vi "Get global var file or mem.vi"(8 "error in (no error)":errorcluster, 9 "Config file path name":string="use default", 10 "Key Name":string="test_pc_name", 11 "Section Name":string="general") -> (0 "error out":errorcluster, 1 "Yes?":bool, 2 "KeyFound?":bool, 3 "Key data from file":string)   [LabVIEW 2013]
doc: "Gets key data from global.ini file in exe directory"
uses:
  <vilib>/Utility/error.llb/whitespace.ctl
  Test Globals/Global 1.vi
panel:
  out "Boolean":bool
  out "Using memory?":bool
  out "Info block":string
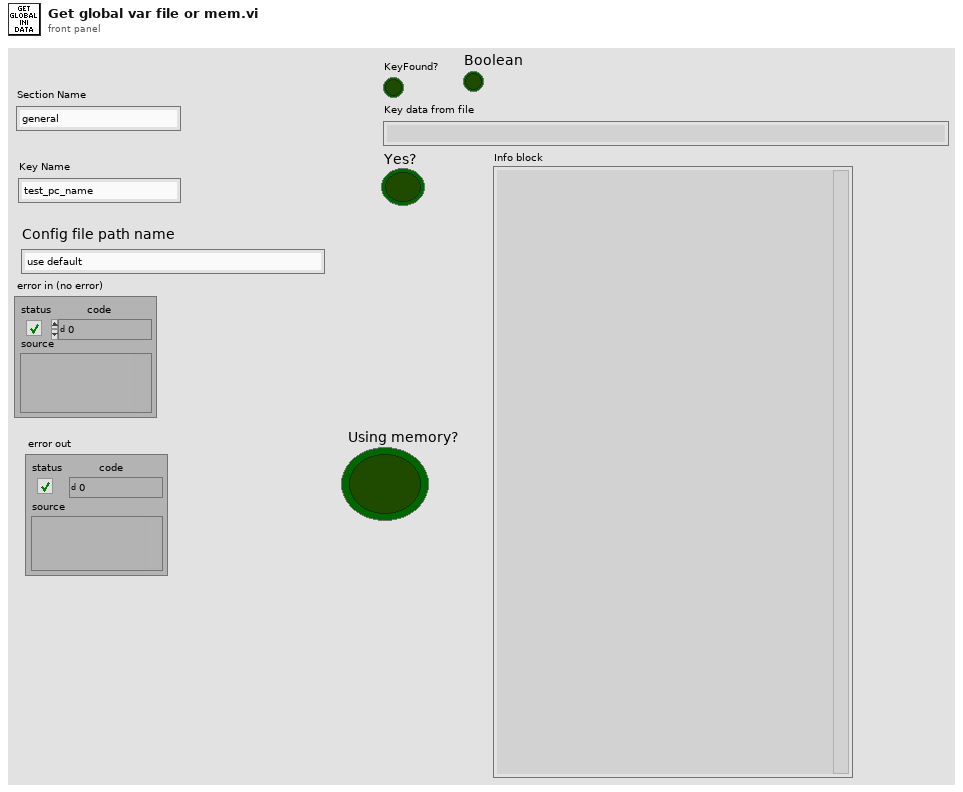
[diagram p1: front panel]
types:
  T1 = cluster{"Test folder":string, "Top level":string, "Main":string, "Test report":string, "Work order qty":string, "Work order meid":string, "Work order imei":string, "Master meid imei list":string, "Master test data":string, "ZPL label info":string, "Pictures":string, "Setup info":string, "Work order":string, "Tests folder":string, "Tests steps folder":string, "Config folder":string, "Verizon Upload file":string, "Job data file":string, "Station globals":string, "Post test info":string}
  T2 = typedef "whitespace.ctl" = u16
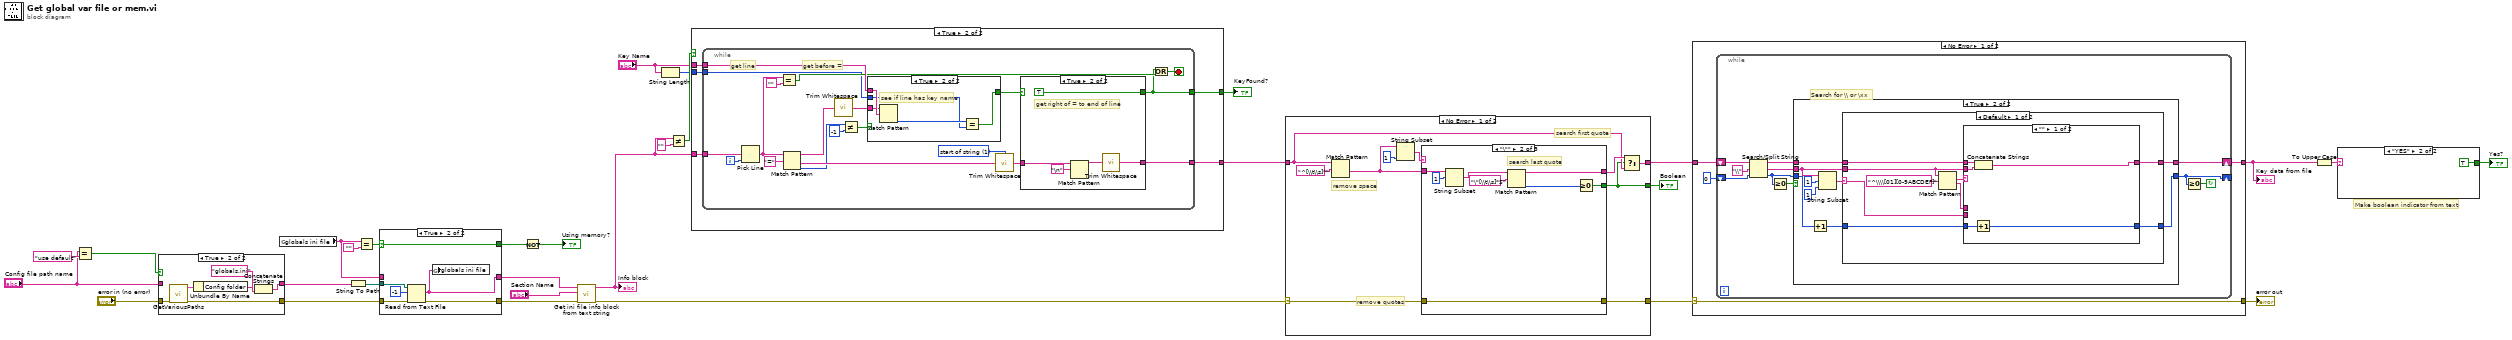
[diagram p0: block diagram]
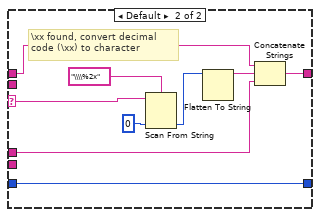
[diagram p4: hidden frame]
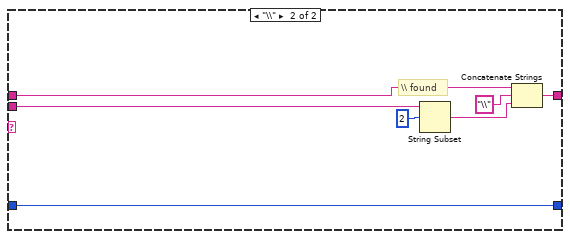
[diagram p5: hidden frame]
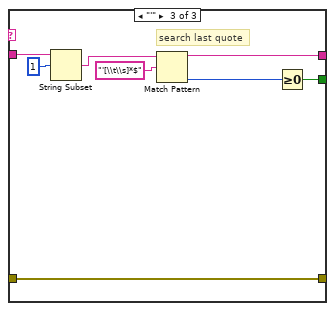
[diagram p8: hidden frame]
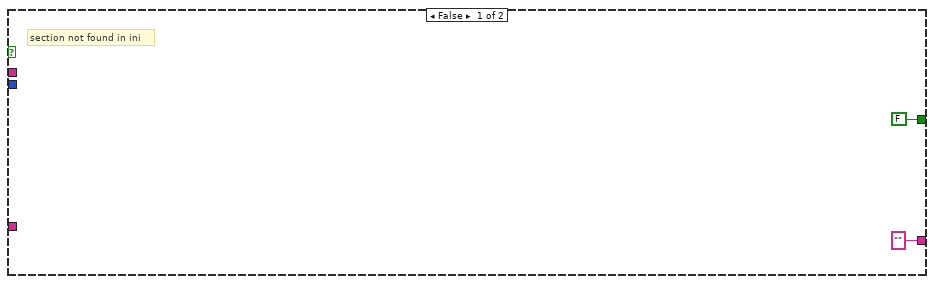
[diagram p10: hidden frame]
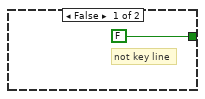
[diagram p11: hidden frame]
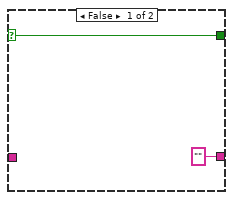
[diagram p12: hidden frame]
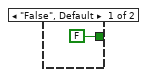
[diagram p14: hidden frame]
diagram:
  # "Make boolean indicator from text"
  n1 = Equal?(x="Config file path name", y="use default") -> (x = y?=w2:bool)
  n2 = case shown="True" w2 {
    tunnel: "error in (no error)" -> [w31 w35]
    tunnel: [w32 w34] -> w29
    tunnel: [w31 w33] -> w24
    tunnel: "Config file path name" -> [w32 _]
    frame False {
    }
    frame True {
      n3 = call "GetVariousPaths.vi"("error in (no error)"=w35) -> ("error out"=w33:errorcluster, "Built Paths"=w37:T1)  [unwired: 9 in]
      n4 = Unbundle By Name(w37) -> ("Config folder"=w36:string)
      n5 = Concatenate Strings(w36, "globals.ini" ("string")) -> (w34:string)
    }
  }
  n6 = global read "Global 1.vi" "globals ini file"() -> (w22:string)
  n7 = String To Path(string=w29) -> (path=w4:path)
  n8 = Equal?(x=w22, y="") -> (x = y?=w25:bool)
  n9 = case shown="True" w25 {
    selector: w25 -> [w39 w44]
    tunnel: w24 -> [w40 w47]
    tunnel: [w40 w46] -> w21
    tunnel: [w41 w42] -> w23
    tunnel: w22 -> [w41 _]
    tunnel: [w39 w44] -> w12
    tunnel: w4 -> [_ w43]
    frame False {
    }
    frame True {
      n10 = Read from Text File(file (use dialog)=w43, count=-1, error in=w47) -> (text=w42:string, error out=w46:errorcluster)  [unwired: 1 in, 2 out]
      n11 = global write "Global 1.vi" "globals ini file"(w42) -> ()
    }
  }
  n12 = Not(x=w12) -> (.not. x?=→"Using memory?":bool)
  n13 = call "Get ini file info block from text string.vi"("error in (no error)"=w21, "Section key"="Section Name", "String"=w23) -> ("error out"=w10:errorcluster, "Info block"=w17:string)  [unwired: 6 in, 1 out]
  "Info block" <- w17
  n14 = String Length(string="Key Name") -> (length=w15:i32)
  n15 = Not Equal?(x=w17, y="") -> (x != y?=w18:bool)
  n16 = case shown="True" w18 {
    tunnel: w17 -> [_ w54]
    tunnel: "Key Name" -> [_ w53]
    tunnel: ["" ("trimmed string") w52] -> w11
    tunnel: w15 -> [_ w51]
    tunnel: [FALSE w50] -> w14
    frame False {
      # "section not found in ini"
    }
    frame True {
      n17 = while {
        tunnel: w54 -> [w74]
        tunnel: w53 -> [w72]
        tunnel: [w70] -> w52
        tunnel: w51 -> [w56]
        tunnel: [w55] -> w50
        i -> [w73]
        stop <- w69 stop-if-true
        w62 = T2 1 items=["both", "start of string", "end of string"] ("location (both)")
        # "get before ="
        # "get line"
        n18 = Pick Line(multi-line string=w74, line index=w73) -> (output string=w65:string)  [unwired: 1 in]
        n19 = Equal?(x=w65, y="") -> (x = y?=w68:bool)
        n20 = Match Pattern(string=w65, regular expression="=") -> (before substring=w64:string, after substring=w63:string, offset past match=w60:i32)  [unwired: 1 in, 1 out]
        n21 = call <vilib>:"Trim Whitespace.vi"("string"=w64) -> ("trimmed string"=w57:string)  [unwired: 1 in]
        n22 = Not Equal?(x=w60, y=-1) -> (x != y?=w58:bool)
        n23 = case shown="True" w58 {
          tunnel: w72 -> [_ w80]
          tunnel: [FALSE w78] -> w71
          tunnel: w57 -> [_ w77]
          tunnel: w56 -> [_ w76]
          frame False {
            # "not key line"
          }
          frame True {
            # "see if line has key name"
            n24 = Match Pattern(string=w77, regular expression=w80) -> (offset past match=w79:i32)  [unwired: 1 in, 3 out]
            n25 = Equal?(x=w79, y=w76) -> (x = y?=w78:bool)
          }
        }
        n26 = call <vilib>:"Trim Whitespace.vi"("string"=w63, "location (both)"=w62) -> ("trimmed string"=w61:string)
        n27 = case shown="True" w71 {
          selector: w71 -> [w81 _]
          tunnel: ["" ("trimmed string") w87] -> w70
          tunnel: [w81 TRUE] -> w55
          tunnel: w61 -> [_ w85]
          frame False {
          }
          frame True {
            # "get right of = to end of line"
            n28 = Match Pattern(string=w85, regular expression="\n") -> (before substring=w84:string)  [unwired: 1 in, 3 out]
            n29 = call <vilib>:"Trim Whitespace.vi"("string"=w84) -> ("trimmed string"=w87:string)  [unwired: 1 in]
          }
        }
        n30 = Or(x=w55, y=w68) -> (x .or. y?=w69:bool)
      }
    }
  }
  "KeyFound?" <- w14
  n31 = case shown="No Error" w10 {
    selector: w10 -> [w88 w116]
    tunnel: [w91 w115] -> w8
    tunnel: w11 -> [w92 w115]
    tunnel: [w89 w116] -> w9
    tunnel: [w90 _] -> w7
    frame No Error {
      # "remove quotes"
      # "remove space"
      # "search first quote"
      n32 = Match Pattern(string=w92, regular expression="^[\\t\\s]*") -> (after substring=w97:string)  [unwired: 1 in, 3 out]
      n33 = String Subset(string=w97, length (rest)=1 ("length (rest)")) -> (substring=w95:string)  [unwired: 1 in]
      n34 = case shown="\"\\\"\"" w95 {
        tunnel: [_ w105 w112] -> w90
        tunnel: [_ w104 w113] -> w96
        tunnel: w97 -> [_ w102 w110]
        tunnel: w88 -> [w98 w100 w108]
        tunnel: [w98 w100 w108] -> w89
        frame Default {
        }
        frame "\"" {
          # "search last quote"
          n35 = String Subset(string=w102, offset (0)=1 ("length (rest)")) -> (substring=w101:string)  [unwired: 1 in]
          n36 = Match Pattern(string=w101, regular expression="\"[\\t\\s]*$") -> (before substring=w104:string, offset past match=w99:i32)  [unwired: 1 in, 2 out]
          n37 = Greater Or Equal To 0?(x=w99) -> (x >= 0?=w105:bool)
        }
        frame "'" {
          # "search last quote"
          n38 = String Subset(string=w110, offset (0)=1 ("length (rest)")) -> (substring=w109:string)  [unwired: 1 in]
          n39 = Match Pattern(string=w109, regular expression="'[\\t\\s]*$") -> (before substring=w113:string, offset past match=w107:i32)  [unwired: 1 in, 2 out]
          n40 = Greater Or Equal To 0?(x=w107) -> (x >= 0?=w112:bool)
        }
      }
      n41 = Select(t=w96, s=w90, f=w92) -> (s? t:f=w91:string)
    }
    frame Error {
    }
  }
  "Boolean" <- w7
  n42 = case shown="No Error" w9 {
    selector: w9 -> [w117 w172]
    tunnel: w8 -> [w119 w173]
    tunnel: [w118 w173] -> w5
    tunnel: [w117 w172] -> w6
    frame No Error {
      n43 = while {
        shift-left: 0 -> [w126]
        shift-right: [w128] -> _
        shift-left: w119 -> [w127]
        shift-right: [w130] -> w118
        stop <- w129 continue-if-true
        # "Search for \\\\ or \\xx"
        n44 = Search/Split String(string=w127, search string/char (-)="\\", offset (0)=w126) -> (substring before match=w122:string, match + rest of string=w121:string, offset of match=w123:i32)
        n45 = Greater Or Equal To 0?(x=w123) -> (x >= 0?=w124:bool)
        n46 = case shown="True" w124 {
          tunnel: [w132 w141] -> w130
          tunnel: w123 -> [w131 w136]
          tunnel: [w131 w140] -> w128
          tunnel: w122 -> [w132 w139]
          tunnel: w121 -> [_ w135]
          frame False {
          }
          frame True {
            n47 = Increment(x=w136) -> (x+1=w133:i32)
            n48 = String Subset(string=w135, offset (0)=1, length (rest)=1 ("length (rest)")) -> (substring=w138:string)
            n49 = case shown="Default" w138 {
              selector: w138 -> [w150 _]
              tunnel: [w145 w171] -> w141
              tunnel: w133 -> [w143 w165]
              tunnel: [w144 w165] -> w140
              tunnel: w139 -> [w146 w169]
              tunnel: w135 -> [w147 w168]
              frame Default {
                n50 = Match Pattern(string=w147, regular expression="^\\\\[01][0-9ABCDEF]") -> (match substring=w148:string, after substring=w142:string)  [unwired: 1 in, 2 out]
                n51 = case shown="\"\"" w148 {
                  selector: w148 -> [_ w161]
                  tunnel: w150 -> [_ _]
                  tunnel: w147 -> [w154 _]
                  tunnel: w146 -> [w155 w159]
                  tunnel: [w153 w160] -> w145
                  tunnel: [w151 w156] -> w144
                  tunnel: w143 -> [w152 w156]
                  tunnel: w142 -> [_ w157]
                  frame "" {
                    n52 = Increment(x=w152) -> (x+1=w151:i32)
                    n53 = Concatenate Strings(w155, w154) -> (w153:string)
                  }
                  frame Default {
                    # "\\xx found, convert decimal \ncode (\\xx) to character"
                    n54 = Scan From String(format string="\\\\%2x" ("Input String"), input string=w161, default 1=u8 0) -> (output 1=w163:u8)  [unwired: 2 in, 3 out]
                    n55 = Flatten To String(anything=w163) -> (data string=w158:string)  [unwired: 1 in, 4 out]
                    n56 = Concatenate Strings(w159, w158, w157) -> (w160:string)
                  }
                }
              }
              frame "\\" {
                # "\\\\ found"
                n57 = String Subset(string=w168, offset (0)=2) -> (substring=w166:string)  [unwired: 1 in]
                n58 = Concatenate Strings(w169, "\\" ("Input String"), w166) -> (w171:string)
              }
            }
          }
        }
        n59 = Greater Or Equal To 0?(x=w128) -> (x >= 0?=w129:bool)
      }
    }
    frame Error {
    }
  }
  "Key data from file" <- w5
  "error out" <- w6
  n60 = To Upper Case(1:w5) -> (0:w28:string)
  n61 = case shown="\"YES\"" w28 {
    tunnel: [FALSE TRUE] -> w27
    frame "False", Default {
    }
    frame "YES" {
    }
  }
  "Yes?" <- w27
